vi "Receive Value Change Event.vi"(8 "error in (no error)":errorcluster, 10 "ValueChangeMsg":refnum<class "ValueChangeMsg.lvclass">, 11 "IViewable In":refnum<class "IViewable.lvclass">) -> (0 "error out":errorcluster, 3 "IViewable Out":refnum<class "IViewable.lvclass">)   [LabVIEW 2020, in "IViewable.lvlib" / "IViewable.lvclass"]
doc: "<License>\nCopyright © 2017 Composed Systems, LLC | All rights reserved\nwww.composed.io\n\nAuthor: Ethan Stern <ethan.stern@composed.io>\n\nThis software is provided \"AS IS\" WITHOUT WARRANTIES, either express or implied, AND IS FOR EDUCATIONAL PURPOSES ONLY.\n</License>"
uses:
  <vilib>/gpm_packages/@cs/mva-viewable/Source/IViewable/IViewable/IViewable.lvclass
  C:/Program Files/National Instruments/LabVIEW 2020/vi.lib/ActorFramework/Actor/Actor.lvclass
  <vilib>/gpm_packages/@cs/mva-viewable/Source/ActorEvents/IEventAggregator Messages/ValueChangeMsg/ValueChangeMsg.lvclass
  <vilib>/ActorFramework/Actor/Actor.lvclass/Actor.ctl
  <vilib>/gpm_packages/@cs/mva-viewable/Source/ActorEvents/IEventAggregator Messages/ValueChangeMsg/ValueChangeMsg.lvclass/ValueChangeMsg.ctl
  <vilib>/gpm_packages/@cs/mva-viewable/Source/IViewable/IViewable Messages/Catch Nested Value Change Msg/Nested Value Update Msg.lvclass/Nested Value Update Msg.ctl
  <vilib>/ActorFramework/Message Enqueuer/Message Enqueuer.lvclass/Message Enqueuer.ctl
  <vilib>/ActorFramework/Message Enqueuer/Enqueue.vi
  <vilib>/gpm_packages/@cs/mva-viewable/Source/IViewable/IViewable Messages/Catch Nested Value Change Msg/Nested Value Update Msg.lvclass
  C:/Program Files/National Instruments/LabVIEW 2020/vi.lib/ActorFramework/Message/Message.lvclass
  <vilib>/ActorFramework/Message Priority Queue/Priority Enqueue.vi
  <vilib>/ActorFramework/Actor/Actor.lvclass
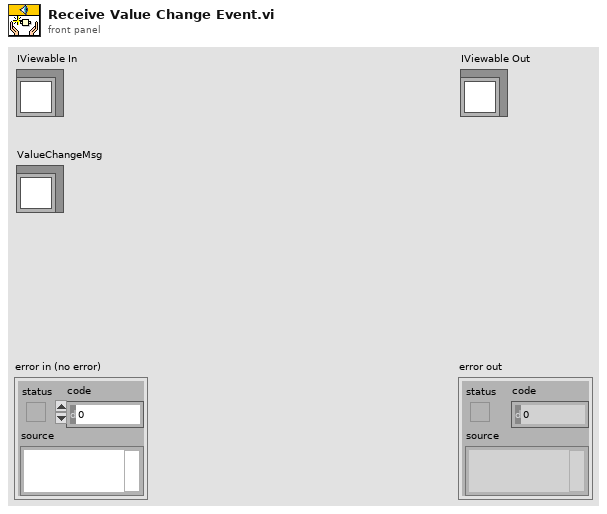
[diagram p1: front panel]
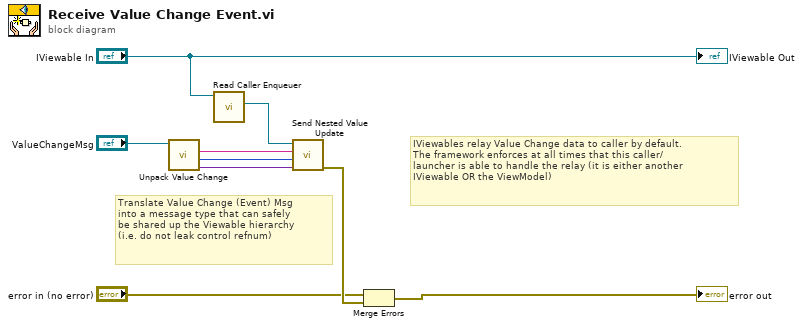
[diagram p0: block diagram]
diagram:
  # "Translate Value Change (Event) Msg\ninto a message type that can safely\nbe shared up the Viewable hierarchy\n(i.e. do not leak control refnum)"
  # "IViewables relay Value Change data to caller by default.\nThe framework enforces at all times that this caller/\nlauncher is able to handle the relay (it is either another\nIViewable OR the ViewModel)"
  n1 = call <vilib>:"Unpack Value Change.vi"("ValueChangeMsg"="ValueChangeMsg") -> ("New Value"=w1:variant, "Time"=w2:u32, "Control Label"=w3:string)  [unwired: 6 in, 2 out]
  n2 = call <vilib>:"Read Caller Enqueuer.vi"("Actor"="IViewable In") -> ("Caller Enqueuer"=w8:refnum<class "Message Enqueuer.lvclass">)  [unwired: 10 in]
  n3 = call <vilib>:"Send Nested Value Update.vi"("Value"=w1, "Time (Get Time)"=w2, "Datum Name"=w3, "Message Enqueuer"=w8) -> ("error out"=w9:errorcluster)  [unwired: 6 in, 1 out]
  n4 = Merge Errors("error in (no error)", w9) -> (→"error out":errorcluster)
  "IViewable Out" <- "IViewable In"
